vi "VariableManager_Double.vi"(7 "Operation":enum16{"Get Tag", "Set Tag"}(ring), 8 "error in (no error)":errorcluster, 10 "Value":dbl, 11 "Tag":string) -> (0 "error out":errorcluster, 2 "Value out":dbl, 3 "Tag Out":string, 4 "Found":bool, 5 "All Tags":cluster{"Tags":string[], "Values":variant[]})   [LabVIEW 2018]
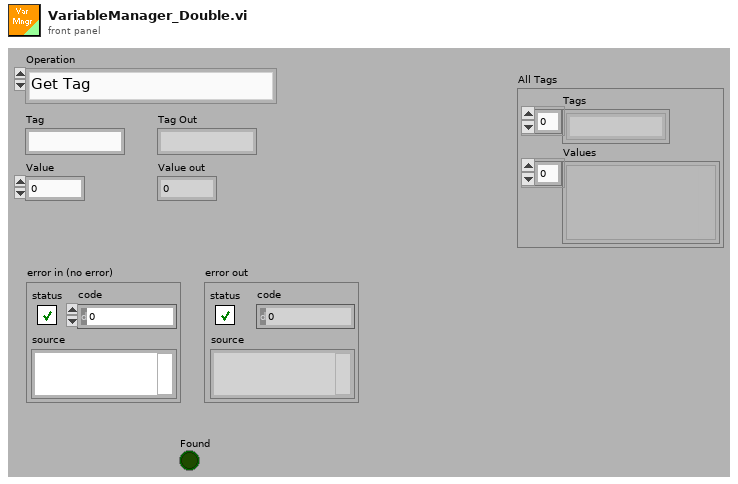
[diagram p1: front panel]
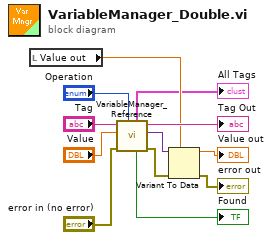
[diagram p0: block diagram]
diagram:
  n1 = local read "Value out"() -> (w5:dbl)
  n2 = call "VariableManager_Reference.vi"("Operation"="Operation", "error in (no error)"="error in (no error)", "Value"="Value", "Tag"="Tag") -> ("error out"=w6:errorcluster, "Value out"=w7:variant, "Tag Out"=→"Tag Out":string, "Found"=→"Found":bool, "All Tags"=→"All Tags":cluster{"Tags":string[], "Values":variant[]})  [unwired: 3 in]
  n3 = Variant To Data(error in=w6, type=w5, Variant=w7) -> (data=→"Value out":dbl, error out=→"error out":errorcluster)
